vi "GetName.vi"(6 "error in":errorcluster, 9 "FlatSequenceFrame in":refnum<class "FlatSequenceFrame.lvclass">) -> (0 "error out":errorcluster, 3 "FlatSequenceFrame out":refnum<class "FlatSequenceFrame.lvclass">, 4 "name":string, 5 "UID":string)   [LabVIEW 2014, in "Raspberry Pi Compatible Compiler for LabVIEW.lvlib" / "FlatSequenceFrame.lvclass"]
uses:
  FlatSequenceFrame.lvclass
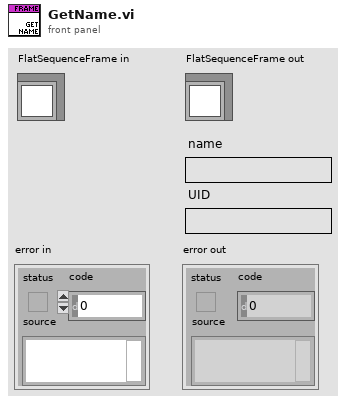
[diagram p1: front panel]
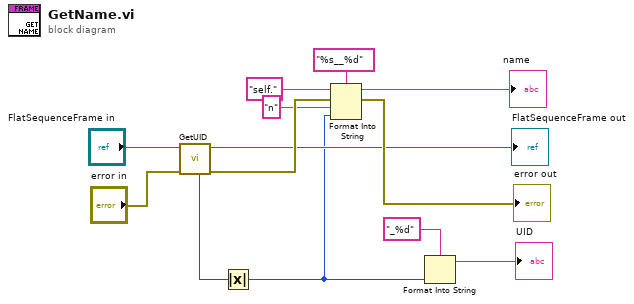
[diagram p0: block diagram]
diagram:
  n1 = call-dynamic "GetUID.vi"("error in"="error in", "FlatSequenceFrame in"="FlatSequenceFrame in") -> ("error out"=w12:errorcluster, "FlatSequenceFrame out"=→"FlatSequenceFrame out":refnum<class "FlatSequenceFrame.lvclass">, "UID"=w4:i32)  [unwired: 5 in]
  n2 = Absolute Value(x=w4) -> (abs(x)=w1:i32)
  n3 = Format Into String(format string="%s__%d", initial string="self." ("format string"), error in=w12, "n" ("input 1"), w1) -> (resulting string=→"name":string, error out=→"error out":errorcluster)
  n4 = Format Into String(format string="_%d", w1) -> (resulting string=→"UID":string)  [unwired: 2 in, 1 out]
